vi "Unregister For Event.vi"(8 "Error In":errorcluster, 9 "Event Name":string, 10 "Registrant Address":refnum<class "Message Enqueuer.lvclass">, 11 "Event Source In":refnum<class "Event Source.lvclass">) -> (0 "Error Out":errorcluster, 3 "Event Source Out":refnum<class "Event Source.lvclass">)   [LabVIEW 2020, in "Event Source.lvlib" / "Event Source.lvclass"]
doc: "This method unregisters a specific Actors Enqueuer from specific Event he is listening to, in this Event Source Actor."
uses:
  Event Source.lvclass
  <vilib>/ActorFramework/Message Enqueuer/Message Enqueuer.lvclass
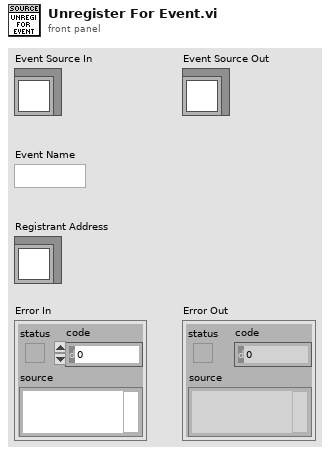
[diagram p1: front panel]
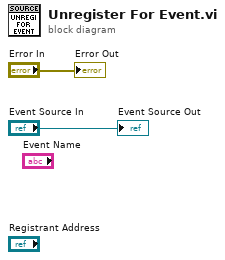
[diagram p0: block diagram]
diagram:
  "Error Out" <- "Error In"
  "Event Source Out" <- "Event Source In"
